vi "Set Item Property (Double).vi"(8 "error in (no error)":errorcluster, 9 "Value":dbl, 10 "Property Name":string, 11 "Item Ref in":T1 format="%.0x") -> (0 "error out":errorcluster, 3 "Item Ref out":T1 format="%.0x", 4 "Replaced":bool)   [LabVIEW 2020, in "Custom Device API.lvlib"]
doc: "Sets a <B>Property Name</B> and <B>Value</B> for an item property and saves this information in the system definition file. If the <B>Property Name</B> you specify already exists, this VI overwrites the property. Wire data to the <B>Value</B> input to determine the polymorphic instance to use or manually select the instance."
uses:
  <vilib>/NI VeriStand/Custom Device API/Custom Device API.lvlib
  <vilib>/NI VeriStand/Custom Device API/Custom Device Item Ref.ctl
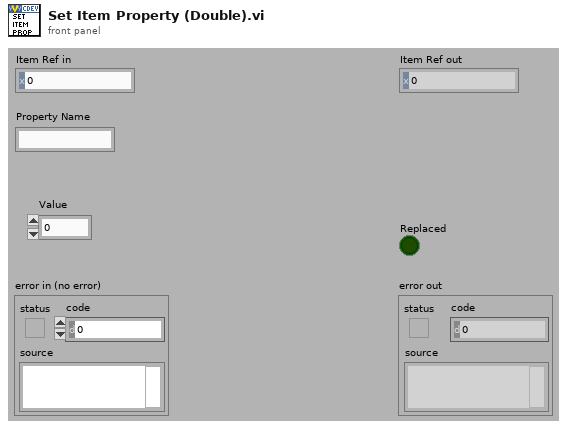
[diagram p1: front panel]
types:
  T1 = typedef "Custom Device API.lvlib/Custom Device Item Ref.ctl" = u64
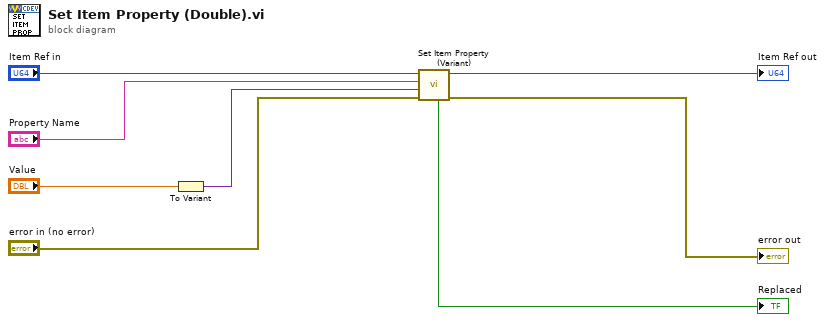
[diagram p0: block diagram]
diagram:
  n1 = To Variant(anything="Value") -> (Variant=w4:variant)
  n2 = call <vilib>:"Set Item Property (Variant).vi"("error in (no error)"="error in (no error)", "Value"=w4, "Property Name"="Property Name", "Item Ref in"="Item Ref in") -> ("error out"=→"error out":errorcluster, "Item Ref out"=→"Item Ref out":T1, "Replaced"=→"Replaced":bool)  [unwired: 5 out]
